vi "GLOBAL_addresses.vi"(9 "Data In":dbl[](array[numeric]), 10 "State":enum16{"Initialise", "Write", "Read"}(ring)) -> (1 "Data out":dbl[](array[numeric]))   [LabVIEW 2014]
panel:
  in  "Index":i32
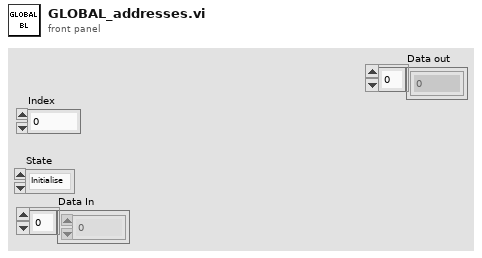
[diagram p1: front panel]
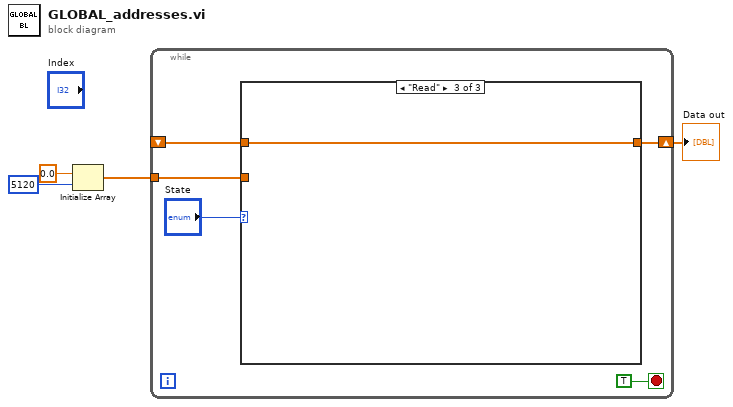
[diagram p0: block diagram]
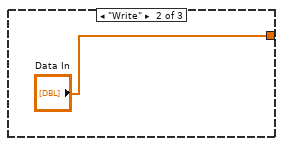
[diagram p3: hidden frame]
diagram:
  n1 = Initialize Array(0.0 ("Numeric"), 5120 ("dimension size")) -> (w2:dbl[])
  n2 = while {
    tunnel: w2 -> [w8]
    shift-right: [w7] -> w1
    shift-left: _ -> [w6]
    stop <- TRUE stop-if-true
    n3 = case shown="\"Read\"" "State" {
      tunnel: w8 -> [w10 _ _]
      tunnel: [w10 "Data In" w12] -> w7
      tunnel: w6 -> [_ _ w12]
      frame "Initialise", Default {
      }
      frame "Write" {
      }
      frame "Read" {
      }
    }
  }
  "Data out" <- w1
